vi "PCO_Open_Struct.vi"() -> (1 "Raw_Length":u16, 4 "Length":u16, 6 "PCO_OpenStruct_Raw_x64":T3, 7 "PCO_OpenStruct_Raw_win32":T1, 8 "PCO_Open_Struct":T2 {"wInterfaceType" format="%x"; "wOpenFlags" format="%x"; "dwOpenFlags" format="%x"})   [LabVIEW 2019, in "SDK.lvlib" / "Structures.lvlib"]
doc: "Use this template to build a VI to use as a subVI."
uses:
  Structures.lvlib
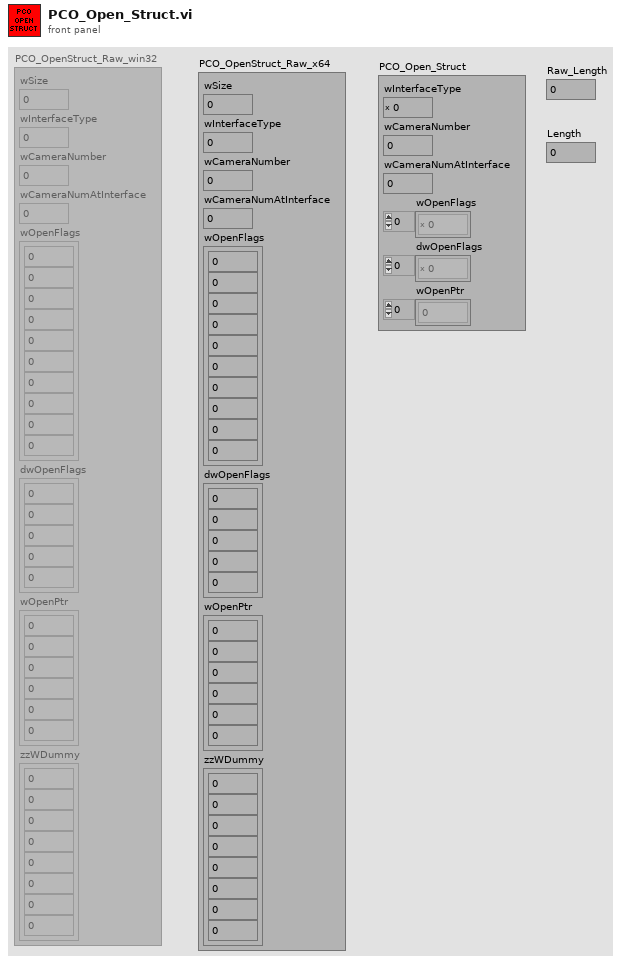
[diagram p1: front panel]
types:
  T1 = cluster{"wSize":u16, "wInterfaceType":u16, "wCameraNumber":u16, "wCameraNumAtInterface":u16, "wOpenFlags":cluster{u16, u16, u16, u16, u16, u16, u16, u16, u16, u16}, "dwOpenFlags":cluster{u32, u32, u32, u32, u32}, "wOpenPtr":cluster{u32, u32, u32, u32, u32, u32}, "zzWDummy":cluster{u16, u16, u16, u16, u16, u16, u16, u16}}
  T2 = cluster{"wInterfaceType":u16, "wCameraNumber":u16, "wCameraNumAtInterface":u16, "wOpenFlags":u16[], "dwOpenFlags":u32[], "wOpenPtr":u64[]}
  T3 = cluster{"wSize":u16, "wInterfaceType":u16, "wCameraNumber":u16, "wCameraNumAtInterface":u16, "wOpenFlags":cluster{u16, u16, u16, u16, u16, u16, u16, u16, u16, u16}, "dwOpenFlags":cluster{u32, u32, u32, u32, u32}, "wOpenPtr":cluster{u64, u64, u64, u64, u64, u64}, "zzWDummy":cluster{u16, u16, u16, u16, u16, u16, u16, u16}}
  T4 = cluster{u16, u16, u16, u16, u16, u16, u16, u16, u16, u16}
  T5 = enum8{"Enabled", "Disabled", "Disabled and Grayed Out"}
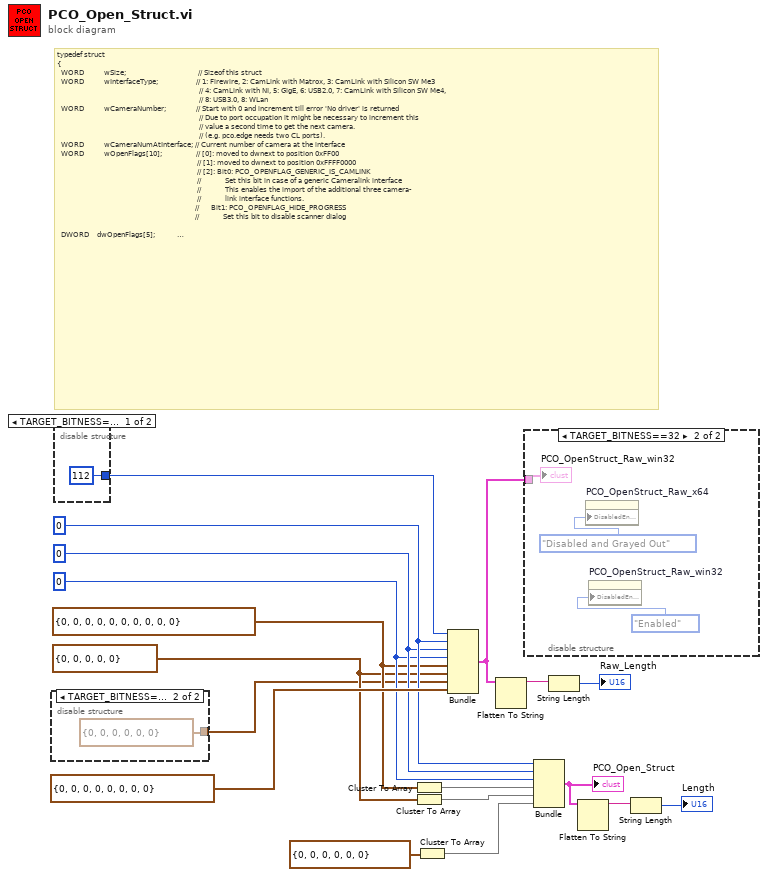
[diagram p0: block diagram]
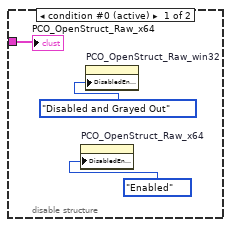
[diagram p2: hidden frame]
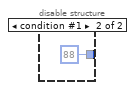
[diagram p3: hidden frame]
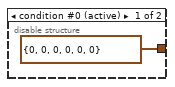
[diagram p4: hidden frame]
diagram:
  w12 = u16 0 ("wCameraNumAtInterface")
  w13 = u16 0 ("wCameraNumber")
  w14 = u16 0 ("wInterfaceType")
  w10 = cluster{u32, u32, u32, u32, u32} {0, 0, 0, 0, 0} ("dwOpenFlags")
  w11 = T4 {0, 0, 0, 0, 0, 0, 0, 0, 0, 0} ("wOpenFlags")
  # "typedef struct\n{\n  WORD          wSize;                                    // Sizeof this struct\n  WORD          wInterfaceType;                   // 1: Firewire, 2: CamLink with Matrox, 3: CamLink with Silicon SW Me3\n                                                                       // 4: CamLink with NI, 5: GigE, 6: USB2.0, 7: CamLink with Silicon SW Me4,\n                                                                       // 8: USB3.0, 8: WLan\n  WORD          wCameraNumber;               // Start with 0 and increment till error 'No driver' is returned\n                                                                       // Due to port occupation it might be necessary to increment this \n                                                                       // value a second time to get the next camera.\n                                                                       // (e.g. pco.edge needs two CL ports).\n  WORD          wCameraNumAtInterface; // Current number of camera at the interface\n  WORD          wOpenFlags[10];                 // [0]: moved to dwnext to position 0xFF00\n                                                                      // [1]: moved to dwnext to position 0xFFFF0000\n                                                                      // [2]: Bit0: PCO_OPENFLAG_GENERIC_IS_CAMLINK\n                                                                      //            Set this bit in case of a generic Cameralink interface\n                                                                      //            This enables the import of the additional three camera-\n                                                                      //            link interface functions.\n                                                                     //      Bit1: PCO_OPENFLAG_HIDE_PROGRESS\n                                                                     //            Set this bit to disable scanner dialog\n\n  DWORD    dwOpenFlags[5];                  // [0]-[4]: moved to strCLOpen.dummy[0]-[4]\n  void*         wOpenPtr[6];\n  WORD      zzwDummy[8];                       // 88 - 64bit: 112\n}PCO_OpenStruct;"
  n1 = disable-structure "Diagram Disable Structure" shown="TARGET_BITNESS==32" {
    disable-tunnel: [cluster{u64, u64, u64, u64, u64, u64} {0, 0, 0, 0, 0, 0} ("wOpenPtr") cluster{u32, u32, u32, u32, u32, u32} {0, 0, 0, 0, 0, 0} ("wOpenPtr")] -> w8
    frame condition #0 (active) {
    }
    frame condition #1 {
    }
  }
  n2 = disable-structure "Diagram Disable Structure" shown="TARGET_BITNESS==64, Default" {
    disable-tunnel: [u16 112 ("wSize") u16 88 ("wSize")] -> w15
    frame condition #0 (active) {
    }
    frame condition #1 {
    }
  }
  n3 = Cluster To Array(cluster=w11) -> (array=w17:u16[])
  n4 = Cluster To Array(cluster=w10) -> (array=w9:u32[])
  n5 = Cluster To Array(cluster=cluster{u64, u64, u64, u64, u64, u64} {0, 0, 0, 0, 0, 0} ("wOpenPtr")) -> (array=w16:u64[])
  n6 = Bundle("wSize"=w15, "wInterfaceType"=w14, "wCameraNumber"=w13, "wCameraNumAtInterface"=w12, "wOpenFlags"=w11, "dwOpenFlags"=w10, "wOpenPtr"=w8, "zzWDummy"=cluster{u16, u16, u16, u16, u16, u16, u16, u16} {0, 0, 0, 0, 0, 0, 0, 0}) -> (w1:T3)  [unwired: 1 in]
  n7 = Flatten To String(anything=w1) -> (data string=w4:string)  [unwired: 3 in, 2 out]
  n8 = disable-structure "Diagram Disable Structure" shown="TARGET_BITNESS==32" {
    disable-tunnel: w1 -> [w25 w28]
    frame condition #0 (active) {
      n9 = property on="PCO_OpenStruct_Raw_x64" class="Clust (strict)"("DisabledEnum"=T5."Enabled" ("Deaktiviert")) -> ()  [unwired: 2 in, 2 out]
      n10 = property on="PCO_OpenStruct_Raw_win32" class="Clust (strict)"("DisabledEnum"=T5."Disabled and Grayed Out" ("Deaktiviert")) -> ()  [unwired: 2 in, 2 out]
      "PCO_OpenStruct_Raw_x64" <- w25
    }
    frame condition #1 {
      n11 = property on="PCO_OpenStruct_Raw_x64" class="Clust (strict)"("DisabledEnum"=T5."Disabled and Grayed Out" ("Deaktiviert")) -> ()  [unwired: 2 in, 2 out]
      n12 = property on="PCO_OpenStruct_Raw_win32" class="Clust (strict)"("DisabledEnum"=T5."Enabled" ("Deaktiviert")) -> ()  [unwired: 2 in, 2 out]
      "PCO_OpenStruct_Raw_win32" <- w28
    }
  }
  n13 = Bundle("wInterfaceType"=w14, "wCameraNumber"=w13, "wCameraNumAtInterface"=w12, "wOpenFlags"=w17, "dwOpenFlags"=w9, "wOpenPtr"=w16) -> (w5:T2)  [unwired: 1 in]
  "PCO_Open_Struct" <- w5
  n14 = String Length(string=w4) -> (length=→"Raw_Length":i32)
  n15 = Flatten To String(anything=w5) -> (data string=w7:string)  [unwired: 3 in, 2 out]
  n16 = String Length(string=w7) -> (length=→"Length":i32)
